vi "Periodic Tasks.vi"(8 "error constant":errorcluster) -> ()   [LabVIEW 2017]
doc: "This VI runs in parallel to other tasks. It can contain as many user-defined periodic loops as you need. These can carry out PID or other sorts of timed response."
uses:
  <vilib>/Rock Robotics/WPI/ThirdParty/Phoenix-LabVIEW/Motor Controller/Controls/CTRE_Phoenix_MotorControl_StatusFrameEnhanced.ctl
  <vilib>/Rock Robotics/WPI/ThirdParty/Phoenix-LabVIEW/Motor Controller/Controls/CTRE_Phoenix_MotorControl_TrajectoryPointTimeDur.ctl
  <vilib>/Rock Robotics/WPI/ThirdParty/Phoenix-LabVIEW/Controls/CTRE_Phoenix_Params.ctl
  <vilib>/Rock Robotics/WPI/ThirdParty/Phoenix-LabVIEW/Motor Controller/Controls/CTRE_Phoenix_MotorControl_ControlMode.ctl
  <vilib>/Rock Robotics/WPI/Utilities/WPI_GetSetVariantRefNum.vi
  Constants.vi
  SelectedMotionProfileMode.vi
  <vilib>/Utility/file.llb/Read Delimited Spreadsheet (DBL).vi
panel:
  out "Mot Prof  Is Under Run":bool
  out "Mot Prof  Has Under Run":bool
  out "Mot Prof Active Is Last":bool
  out "Mot Prof Active Is Valid":bool
  out "Top Mot Prof Count":i32
  out "Mot Prof Active Velocity":dbl
  out "Mot Prof Active Position":dbl
  out "Loop Time":u32
  out "Btm Mot Prof Count":i32
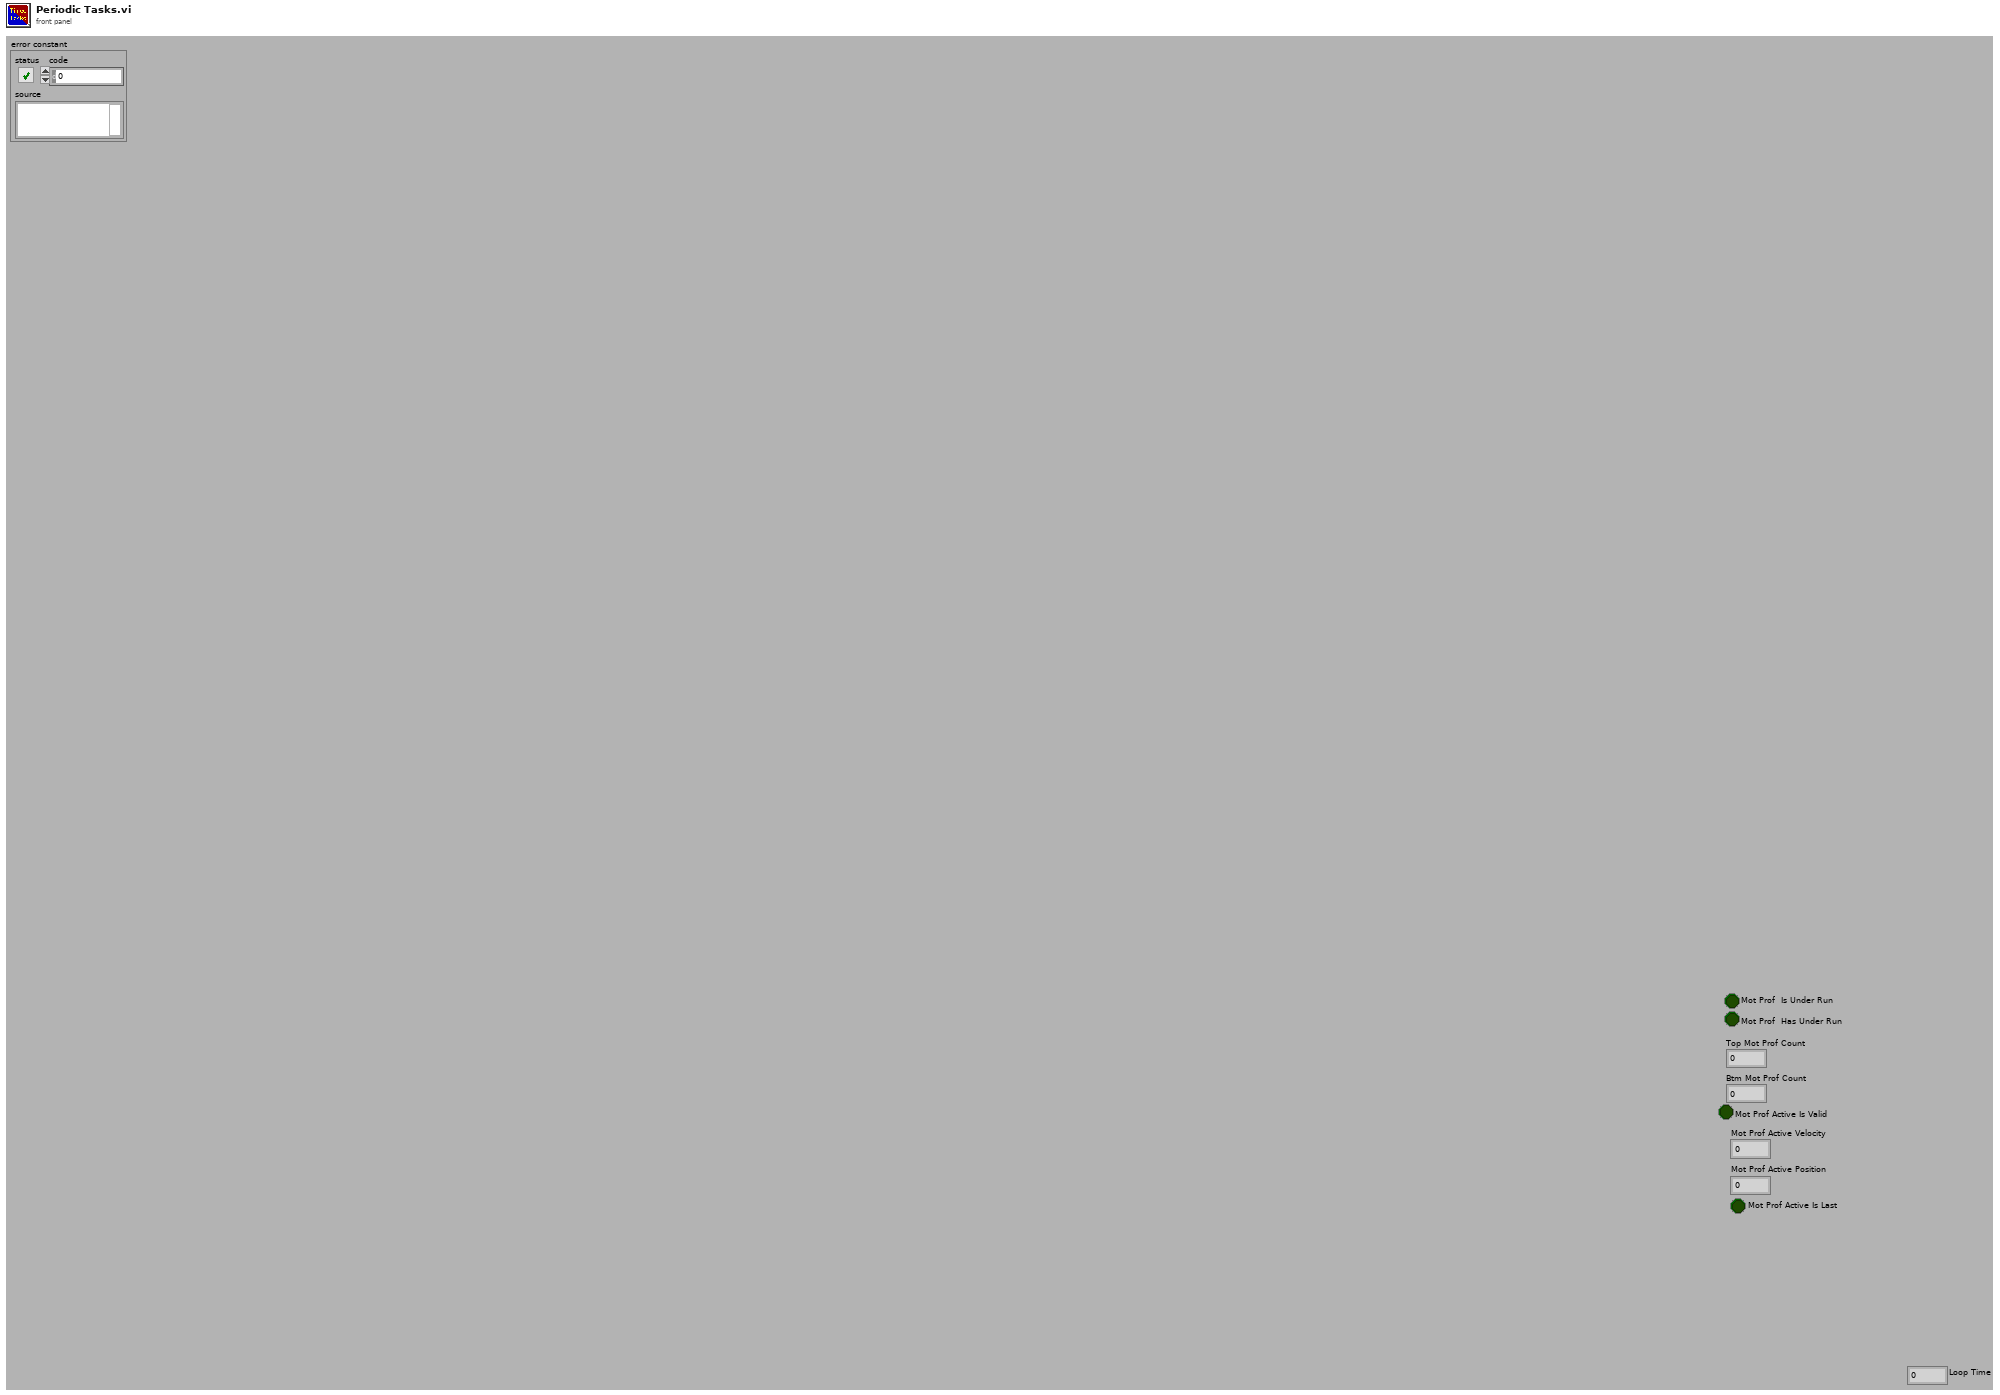
[diagram p1: front panel]
types:
  T1 = typedef "CTRE_Phoenix_MotorControl_StatusFrameEnhanced.ctl" = u16
  T2 = enum16{"One_Axis_PercentOutput", "Two_Axis_PercentOutput", "One_Axix_Position", "One_Axis_Position_CustomFeedFwd", "Two_Axis_Position", "One_Axis_Velocity", "One_Axis_Velocity_CustomFeedFwd", "Two_Axis_Velocity", "One_Axis_MotionMagic", "One_Axis_MotionMagic_CustomFeedFwd", "Two_Axis_MotionMagic", "One_Axis_MotionProfile", "One_Axis_MotionProfile_CustomFeedFwd", "Two_Axis_MotionProfile", "Two_Axis_MotionProfile_CustomFeedFwd"}
  T3 = typedef "WPI_MotorControlDeviceRef.ctl" = cluster{"DeviceStatus":errorcluster, "Type":T4, "PWM":cluster{"PWM Channel":T5, "DeadBand":T6}, "CAN":cluster{"Device Number":u8, "SetOutput VI Ref":variant, "GetOutput VI Ref":variant, "Enable VI Ref":variant, "Disable VI Ref":variant, "Data":variant}, "Invert":bool, "DIO PWM":cluster{"PWM \"Enable\" Channel":T5, "DIOChannel":T7, "PWM Rate":dbl}}
  T4 = typedef "WPI_MotorControlType.ctl" = enum16{"PWM", "CAN", "DIO PWM"}
  T5 = typedef "FPGA_DIOPWMChannel.ctl" = enum8{"PWM 0", "PWM 1", "PWM 2", "PWM 3", "PWM 4", "PWM 5", "PWM 6", "PWM 7", "PWM 8", "PWM 9", "PWM MXP 0", "PWM MXP 1", "PWM MXP 2", "PWM MXP 3", "PWM MXP 4", "PWM MXP 5", "PWM MXP 6", "PWM MXP 7", "PWM MXP 8", "PWM MXP 9", "Invalid"}
  T6 = typedef "WPI_PWMDeadband.ctl" = cluster{"Name":string, "maxPositivePwm":i32, "minPositivePwm":i32, "centerPwm":i32, "maxNegativePwm":i32, "minNegativePwm":i32, "angularRange":u16}
  T7 = typedef "FPGA_DIOChannel.ctl" = enum8{"DIO 0", "DIO 1", "DIO 2", "DIO 3", "DIO 4", "DIO 5", "DIO 6", "DIO 7", "DIO 8", "DIO 9", "DIO MXP 0", "DIO MXP 1", "DIO MXP 2", "DIO MXP 3", "DIO MXP 4", "DIO MXP 5", "DIO MXP 6", "DIO MXP 7", "DIO MXP 8", "DIO MXP 9", "DIO MXP 10", "DIO MXP 11", "DIO MXP 12", "DIO MXP 13", "DIO MXP 14", "DIO MXP 15", "SPI Port CS1", "SPI Port CS2", "SPI Port CS3", "SPI Port MISO", "SPI Port MOSI", "Invalid"}
  T8 = typedef "CTRE_PigeonIMU_DeviceRef.ctl" = cluster{"DeviceStatus":errorcluster, "Device Number":u8, "Type":T9, "Device ID":u32, "Handle":u64, "UsageFrame":u32, "Library Path":path}
  T9 = typedef "CTRE_PigeonIMU_ConnectionType.ctl" = u32
  T10 = typedef "WPI_JoystickDevRef.ctl" = cluster{"Device":T11}
  T11 = typedef "WPI_JoystickDeviceEnum.ctl" = enum16{"USB 0", "USB 1", "USB 2", "USB 3", "USB 4", "USB 5"}
  T12 = enum16{"DemandType_Neutral", "DemandType_AuxPID", "DemandType_ArbitraryFeedForward"}
  T13 = enum16{"FollowerType_PercentOutput", "FollowerType_AuxOutput1"}
  T14 = typedef "CTRE_Phoenix_Params.ctl" = u16
  T15 = typedef "CTRE_Phoenix_MotorControl_ControlMode.ctl" = u16
  T16 = cluster{"Top Buffer Remaining":i32, "Top Buffer Count":i32, "Bottom Buffer Count":i32, "Has Underrun?":bool, "Is Underrun?":bool, "Active Point Valid?":bool, "Is Last?":bool, "Profile Slot Select 0":i32, "Output Enable":i32, "Time Duration (ms)":i32, "Profile Slot Select 1":i32}
  T17 = typedef "CTRE_Phoenix_MotorControl_TrajectoryPointTimeDur.ctl" = i32
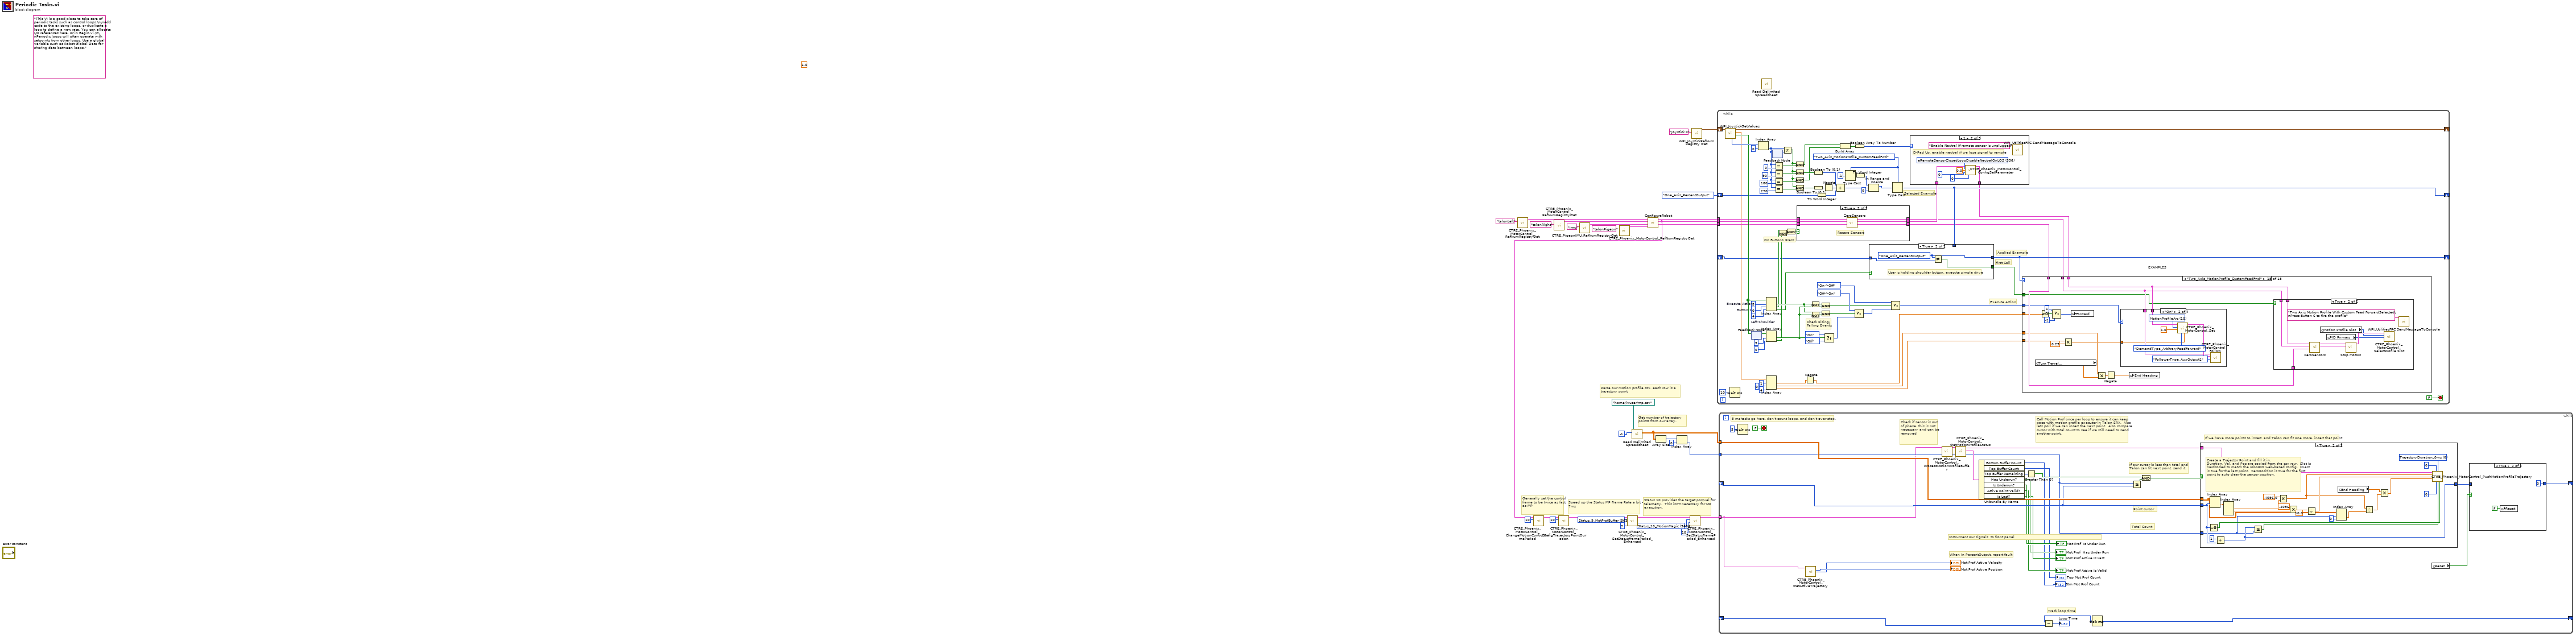
[diagram p0: block diagram]
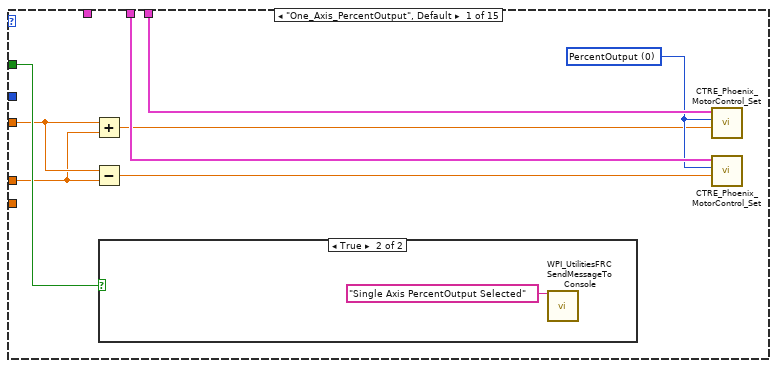
[diagram p4: hidden frame]
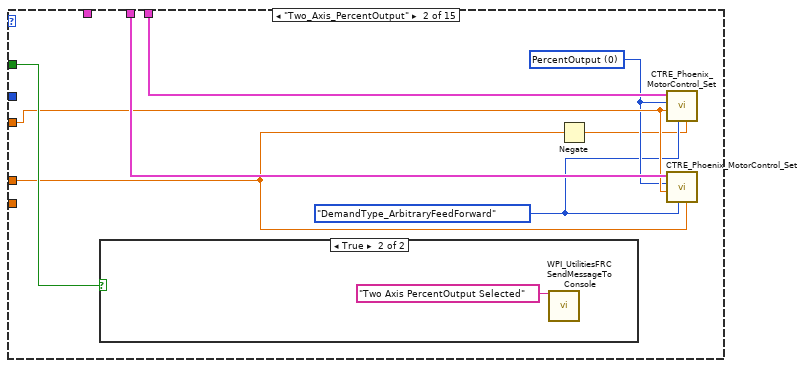
[diagram p6: hidden frame]
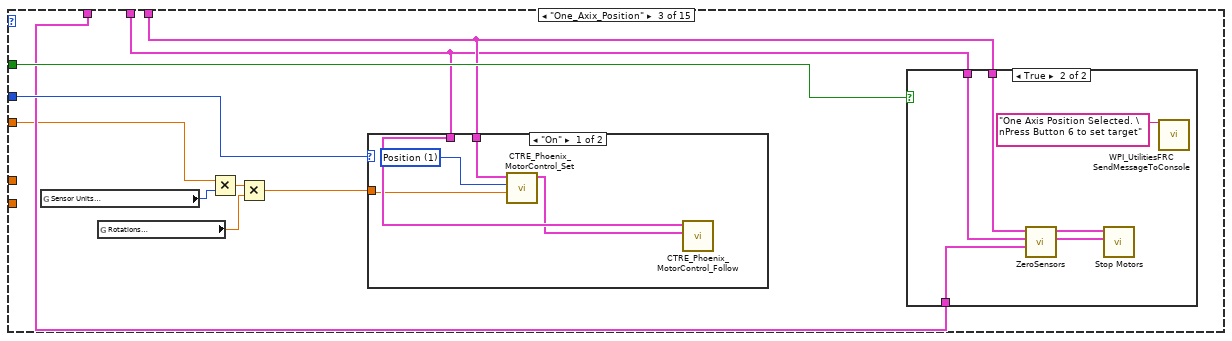
[diagram p8: hidden frame]
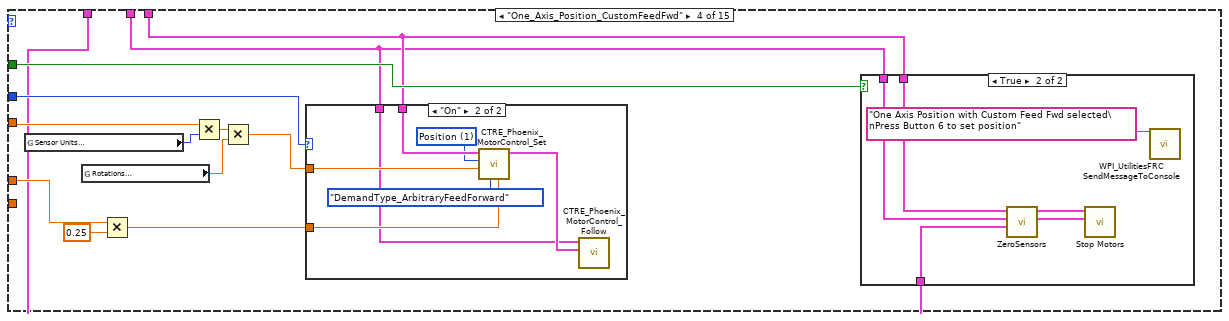
[diagram p11: hidden frame]
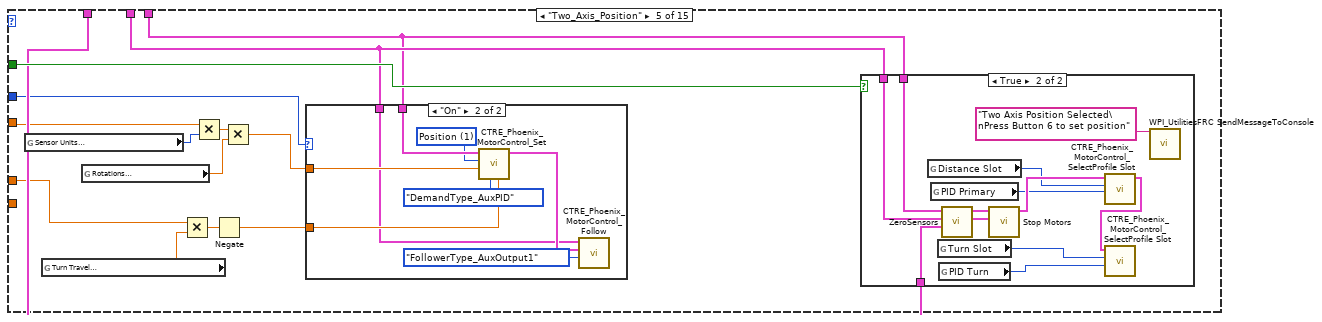
[diagram p14: hidden frame]
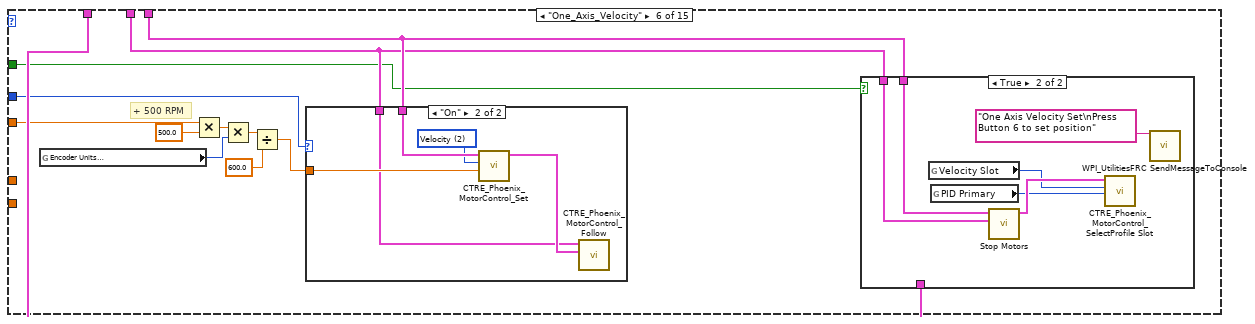
[diagram p17: hidden frame]
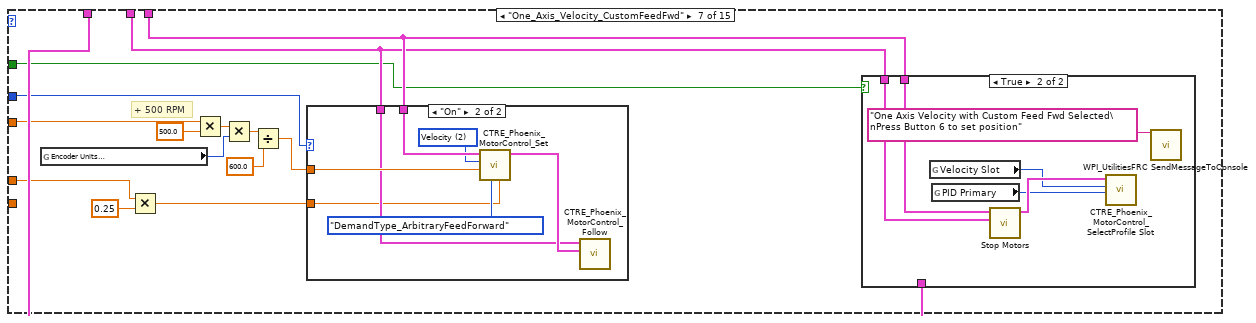
[diagram p20: hidden frame]
diagram:
  w9 = T1 5696 items=["Status_1_General"=5120, "Status_2_Feedback0"=5184, "Status_3_Quadrature"=5248, "Status_4_AinTempVbat"=5312, "Status_6_Misc"=5440, "Status_7_CommStatus"=5504, "Status_8_PulseWidth"=5568, "Status_9_MotProfBuffer"=5632, "Status_10_MotionMagic"=5696, "Status_11_UartGadgeteer"=5760, "Status_12_Feedback1"=5824, "Status_13_Base_PIDF0"=5888, "Status_14_Turn_PIDF1"=5952, "Status_15_FirmwareApiStatus"=6016] ("Status Frame")
  w11 = T1 5632 items=["Status_1_General"=5120, "Status_2_Feedback0"=5184, "Status_3_Quadrature"=5248, "Status_4_AinTempVbat"=5312, "Status_6_Misc"=5440, "Status_7_CommStatus"=5504, "Status_8_PulseWidth"=5568, "Status_9_MotProfBuffer"=5632, "Status_10_MotionMagic"=5696, "Status_11_UartGadgeteer"=5760, "Status_12_Feedback1"=5824, "Status_13_Base_PIDF0"=5888, "Status_14_Turn_PIDF1"=5952, "Status_15_FirmwareApiStatus"=6016] ("Status Frame")
  (unwired) 1.0 ("Forward Peak Percent Output")
  (unwired) "This VI is a good place to take care of periodic tasks such as control loops.\n\nAdd code to the existing loops, or duplicate a loop to define a new rate. You can allocate I/O references here, or in Begin.vi.\n\nPeriodic loops will often operate with setpoints from other loops. Use a global variable such as Robot Global Data for sharing data between loops."
  # "Generally set the control frame to be twice as fast as MP"
  # "Status 10 provides the target pos/vel for telemetry.  This isn't necessary for MP execution."
  # "Speed up the Status MP Frame Rate a bit - 7ms"
  # "Get number of trajectory points from our array."
  # "Parse our motion profile csv, each row is a trajectory point"
  n1 = call <vilib>:"CTRE_Phoenix_MotorControl_RefNumRegistryGet.vi"("refnum name"="talonLeft") -> ("PhoenixMotorControlDevRef"=w23:T3)  [unwired: 9 in, 1 out]
  n2 = call <vilib>:"CTRE_Phoenix_MotorControl_RefNumRegistryGet.vi"("refnum name"="talonRight") -> ("PhoenixMotorControlDevRef"=w24:T3)  [unwired: 9 in, 1 out]
  n3 = call <vilib>:"CTRE_PigeonIMU_RefNumRegistryGet.vi"("refnum name"="imu") -> ("PigeonIMUDevRef"=w19:T8)  [unwired: 9 in, 1 out]
  n4 = call <vilib>:"CTRE_Phoenix_MotorControl_RefNumRegistryGet.vi"("refnum name"="talonPigeon") -> ("PhoenixMotorControlDevRef"=w18:T3)  [unwired: 9 in, 1 out]
  n5 = call-poly <vilib>:"Read Delimited Spreadsheet.vi"("file path (dialog if empty)"=path "/home/lvuser/mp.csv" ("file path (use dialog)"), "number of rows (all:-1)"=-1) -> ("all rows"=w13:dbl[][])  [unwired: 8 in, 5 out]
  n6 = call "ConfigureRobot.vi"("Pigeon Talon"=w18, "Pigeon"=w19, "Right Side"=w24, "Left Side"=w23) -> ("Pigeon"=w20:T8, "Right Side"=w4:T3, "Left Side"=w21:T3)  [unwired: 5 in]
  n7 = call <vilib>:"CTRE_Phoenix_MotorControl_ChangeMotionControlFramePeriod.vi"("periodMs"=10, "PhoenixMotorControlDevRef"=w4) -> ("PhoenixMotorControlDevRef"=w3:T3)  [unwired: 8 in, 1 out]
  n8 = call <vilib>:"CTRE_Phoenix_MotorControl_ConfigTrajectoryPointDuration.vi"("durationMs"=10, "PhoenixMotorControlDevRef"=w3) -> ("PhoenixMotorControlDevRef"=w2:T3)  [unwired: 8 in, 1 out]
  n9 = call <vilib>:"CTRE_Phoenix_MotorControl_SetStatusFramePeriod_Enhanced.vi"("periodMs"=7, "Status Frame"=w11, "PhoenixMotorControlDevRef"=w2) -> ("PhoenixMotorControlDevRef"=w7:T3)  [unwired: 7 in, 1 out]
  n10 = Array Size(array=w13) -> (size(s)=w14:i32[])
  n11 = Index Array(array=w14, index=0) -> (element=w12:i32)
  n12 = call <vilib>:"CTRE_Phoenix_MotorControl_SetStatusFramePeriod_Enhanced.vi"("periodMs"=10, "Status Frame"=w9, "PhoenixMotorControlDevRef"=w7) -> ("PhoenixMotorControlDevRef"=w5:T3)  [unwired: 7 in, 1 out]
  n13 = call <vilib>:"WPI_JoystickRefNum Registry Get.vi"("refnum name"="Joystick 0") -> ("JoystickDevRef"=w29:T10)  [unwired: 1 in, 9 out]
  n14 = while {
    shift-right: [w106] -> _
    shift-left: w29 -> [w107]
    shift-right: [w56] -> _
    shift-left: T2."One_Axis_PercentOutput" -> [w55]
    tunnel: w21 -> [w70]
    tunnel: w4 -> [w69]
    tunnel: w20 -> [w68]
    shift-right: [w57] -> _
    shift-left: _ -> [w58]
    stop <- FALSE stop-if-true
    w49 = T2."Two_Axis_MotionProfile_CustomFeedFwd"
    w60 = 4  # Left Shoulder
    w66 = 0  # Button 1
    w84 = 5  # Execute Action
    # "Execute Action"
    # "Check Rising/\nFalling Events"
    # "First Call"
    # "Applied Example"
    # "On Button1 Press"
    # "Selected Example"
    n15 = call <vilib>:"WPI_JoystickGetValues.vi"("JoystickDevRef"=w107) -> ("Buttons"=w86:bool[], "Axes"=w44:dbl[], "JoystickDevRef"=w106:T10, "POVs"=w105:i16[])  [unwired: 6 in, 1 out]
    n16 = Wait (ms)(milliseconds to wait=u32 10) -> ()  [unwired: 1 out]
    n17 = feedback #1() -> (w85:bool[])  [unwired: 1 in]
    n18 = feedback-in #1(w86) -> ()
    n19 = Index Array(array=w105, index=0) -> (element=w98:i16)
    n20 = Index Array(array=w86, index #1=w84, index #2=w66, index #3=w60) -> (element #1=w77:bool, element #2=w63:bool, element #3=w59:bool)
    n21 = Index Array(array=w85, index #1=5 ("index"), index #2=0 ("index")) -> (element #1=w78:bool, element #2=w61:bool)
    n22 = Index Array(array=w44, index #1=1 ("index"), index #2=0 ("index"), index #3=4 ("index")) -> (element #1=w32:dbl, element #2=w41:dbl, element #3=w33:dbl)
    n23 = feedback #2() -> (w99:i16)  [unwired: 1 in]
    n24 = feedback-in #2(w98) -> ()
    n25 = Equal?(x=w98, y=i16 0) -> (x = y?=w97:bool)
    n26 = Equal?(x=w98, y=i16 90) -> (x = y?=w96:bool)
    n27 = Equal?(x=w98, y=i16 180) -> (x = y?=w95:bool)
    n28 = Equal?(x=w98, y=i16 270) -> (x = y?=w94:bool)
    n29 = Not(x=w61) -> (.not. x?=w62:bool)
    n30 = Not Equal?(x=w98, y=w99) -> (x != y?=w93:bool)
    n31 = And(x=w63, y=w62) -> (x .and. y?=w64:bool)
    n32 = And(x=w93, y=w97) -> (x .and. y?=w88:bool)
    n33 = And(x=w93, y=w96) -> (x .and. y?=w91:bool)
    n34 = And(x=w93, y=w95) -> (x .and. y?=w87:bool)
    n35 = And(x=w93, y=w94) -> (x .and. y?=w92:bool)
    n36 = case shown="True" w64 {
      tunnel: w70 -> [w542 w544]
      tunnel: w69 -> [w543 w545]
      tunnel: w68 -> [w541 w546]
      tunnel: [w543 w548] -> w67
      tunnel: [w542 w549] -> w40
      tunnel: [w541 w547] -> w35
      frame False {
        # "Do Nothing"
      }
      frame True {
        # "Rezero Sensors"
        n37 = call "ZeroSensors.vi"("Pigeon"=w546, "Talon 2"=w545, "Talon 1"=w544) -> ("Pigeon"=w547:T8, "Talon 2"=w548:T3, "Talon 1"=w549:T3)  [unwired: 6 in]
      }
    }
    n38 = Negate(x=w32) -> (-x=w31:dbl)
    n39 = Not(x=w77) -> (.not. x?=w79:bool)
    n40 = Not(x=w78) -> (.not. x?=w80:bool)
    n41 = Boolean To (0,1)(Boolean=w91) -> (0, 1=w38:i16)
    n42 = Boolean To (0,1)(Boolean=w92) -> (0, 1=w36:i16)
    n43 = To Word Integer(number=w55) -> (16bit integer=w54:i16)
    n44 = And(x=w79, y=w78) -> (x .and. y?=w71:bool)
    n45 = And(x=w77, y=w80) -> (x .and. y?=w72:bool)
    n46 = Negate(x=w36) -> (-x=w37:i16)
    n47 = Select(t=enum16{"Off->On", "On->Off", "On", "Off"}."On", s=w78, f=enum16{"Off->On", "On->Off", "On", "Off"}."Off") -> (s? t:f=w76:enum16{"Off->On", "On->Off", "On", "Off"})
    n48 = Compound Arithmetic op=ADD(w38, w37, w54) -> (w53:i16)
    n49 = Build Array(w88, w87) -> (w89:bool[])
    n50 = Type Cast(type=w49, x=i16 -1 ("lower limit")) -> (*(type *) &x=w47:T2)
    n51 = Select(t=enum16{"Off->On", "On->Off", "On", "Off"}."Off->On", s=w72, f=w76) -> (s? t:f=w75:enum16{"Off->On", "On->Off", "On", "Off"})
    n52 = Boolean Array To Number(Boolean array=w89) -> (number=w90:u32)
    n53 = To Word Integer(number=w47) -> (16bit integer=w48:i16)
    n54 = In Range and Coerce(upper limit=w48, x=w53, lower limit=i16 0) -> (coerced(x)=w51:i16)  [unwired: 1 out]
    n55 = Select(t=enum16{"Off->On", "On->Off", "On", "Off"}."On->Off", s=w71, f=w75) -> (s? t:f=w45:enum16{"Off->On", "On->Off", "On", "Off"})
    n56 = Type Cast(type=w49, x=w51) -> (*(type *) &x=w56:T2)
    n57 = case shown="True" w59 {
      tunnel: w58 -> [w535 w540]
      tunnel: [w537 w539] -> w46
      tunnel: [w536 w538] -> w57
      tunnel: w56 -> [w536 _]
      frame False {
        # "User is not holding shoulder button, use applied example"
        n58 = Not Equal?(x=w536, y=w535) -> (x != y?=w537:bool)
      }
      frame True {
        w538 = T2."One_Axis_PercentOutput"
        # "User is holding shoulder button, execute simple drive"
        n59 = Not Equal?(x=w538, y=w540) -> (x != y?=w539:bool)
      }
    }
    n60 = case shown="1" w90 {
      tunnel: w67 -> [w550 w552 w564]
      tunnel: [w550 w553 w563] -> w39
      frame 0, Default {
        # "Nothing Pressed"
      }
      frame 1 {
        w557 = T14 336 items=["eOnBoot_BrakeMode"=31, "eQuadFilterEn"=91, "eQuadIdxPolarity"=108, "eClearPositionOnIdx"=100, "eMotionProfileHasUnderrunErr"=119, "eMotionProfileTrajectoryPointDurationMs"=120, "eClearPosOnLimitF"=144, "eClearPosOnLimitR"=145, "eStatusFramePeriod"=300, "eOpenLoopRamp"=301, "eClosedLoopRamp"=302, "eNeutralDeadband"=303, "ePeakPosOutput"=305, "eNominalPosOutput"=306, "ePeakNegOutput"=307, "eNominalNegOutput"=308, "eProfileParamSlot_P"=310, "eProfileParamSlot_I"=311, "eProfileParamSlot_D"=312, "eProfileParamSlot_F"=313, "eProfileParamSlot_IZone"=314, "eProfileParamSlot_AllowableErr"=315, "eProfileParamSlot_MaxIAccum"=316, "eClearPositionOnLimitF"=320, "eClearPositionOnLimitR"=321, "eClearPositionOnQuadIdx"=322, "eSampleVelocityPeriod"=325, "eSampleVelocityWindow"=326, "eFeedbackSensorType"=330, "eSelectedSensorPosition"=331, "eFeedbackNotContinuous"=332, "eRemoteSensorSource"=333, "eRemoteSensorDeviceID"=334, "eSensorTerm"=335, "eRemoteSensorClosedLoopDisableNeutralOnLOS"=336, "eForwardSoftLimitThreshold"=340, "eReverseSoftLimitThreshold"=341, "eForwardSoftLimitEnable"=342, "eReverseSoftLimitEnable"=343, "eNominalBatteryVoltage"=350, "eBatterVoltageFilterSize"=351, "eContinuousCurrentLimitAmps"=360, "eContinuousCurrentLimitMs"=361, "ePeakCurrentLimitAmps"=362, "eClosedLoopIAccum"=370, "eCustomParam"=380, "eStickyFaults"=390, "eAnalogPosition"=400, "eQuadraturePosition"=401, "ePulseWidthPosition"=402, "eMotMag_Accel"=410, "eMotMag_VelCruise"=411, "eLimitSwitchSource"=421, "eLimitSwitchNormClosedAndDis"=422, "eLimitSwitchDisabledNeutralOnLOS"=423, "eLimitSwitchRemoteDevID"=424] ("Parameter")
        # "D-Pad Up, enable neutral if we lose signal to remote"
        n61 = call <vilib>:"CTRE_Phoenix_MotorControl_ConfigSetParameter.vi"("PhoenixMotorControlDevRef"=w552, "Parameter"=w557, "value"=0.0, "subValue"=u8 0, "ordinal"=0) -> ("PhoenixMotorControlDevRef"=w553:T3)  [unwired: 9 in, 1 out]
        n62 = call <vilib>:"WPI_UtilitiesFRC SendMessageToConsole.vi"("Message"="Enable Neutral if remote sensor is unplugged") -> ()  [unwired: 14 in, 1 out]
      }
      frame 2 {
        w562 = T14 336 items=["eOnBoot_BrakeMode"=31, "eQuadFilterEn"=91, "eQuadIdxPolarity"=108, "eClearPositionOnIdx"=100, "eMotionProfileHasUnderrunErr"=119, "eMotionProfileTrajectoryPointDurationMs"=120, "eClearPosOnLimitF"=144, "eClearPosOnLimitR"=145, "eStatusFramePeriod"=300, "eOpenLoopRamp"=301, "eClosedLoopRamp"=302, "eNeutralDeadband"=303, "ePeakPosOutput"=305, "eNominalPosOutput"=306, "ePeakNegOutput"=307, "eNominalNegOutput"=308, "eProfileParamSlot_P"=310, "eProfileParamSlot_I"=311, "eProfileParamSlot_D"=312, "eProfileParamSlot_F"=313, "eProfileParamSlot_IZone"=314, "eProfileParamSlot_AllowableErr"=315, "eProfileParamSlot_MaxIAccum"=316, "eClearPositionOnLimitF"=320, "eClearPositionOnLimitR"=321, "eClearPositionOnQuadIdx"=322, "eSampleVelocityPeriod"=325, "eSampleVelocityWindow"=326, "eFeedbackSensorType"=330, "eSelectedSensorPosition"=331, "eFeedbackNotContinuous"=332, "eRemoteSensorSource"=333, "eRemoteSensorDeviceID"=334, "eSensorTerm"=335, "eRemoteSensorClosedLoopDisableNeutralOnLOS"=336, "eForwardSoftLimitThreshold"=340, "eReverseSoftLimitThreshold"=341, "eForwardSoftLimitEnable"=342, "eReverseSoftLimitEnable"=343, "eNominalBatteryVoltage"=350, "eBatterVoltageFilterSize"=351, "eContinuousCurrentLimitAmps"=360, "eContinuousCurrentLimitMs"=361, "ePeakCurrentLimitAmps"=362, "eClosedLoopIAccum"=370, "eCustomParam"=380, "eStickyFaults"=390, "eAnalogPosition"=400, "eQuadraturePosition"=401, "ePulseWidthPosition"=402, "eMotMag_Accel"=410, "eMotMag_VelCruise"=411, "eLimitSwitchSource"=421, "eLimitSwitchNormClosedAndDis"=422, "eLimitSwitchDisabledNeutralOnLOS"=423, "eLimitSwitchRemoteDevID"=424] ("Parameter")
        # "D-Pad Up, disable neutral if we lose signal to remote"
        n63 = call <vilib>:"CTRE_Phoenix_MotorControl_ConfigSetParameter.vi"("PhoenixMotorControlDevRef"=w564, "Parameter"=w562, "value"=1.0, "subValue"=u8 0, "ordinal"=0) -> ("PhoenixMotorControlDevRef"=w563:T3)  [unwired: 9 in, 1 out]
        n64 = call <vilib>:"WPI_UtilitiesFRC SendMessageToConsole.vi"("Message"="Disable Neutral if remote sensor is unplugged") -> ()  [unwired: 14 in, 1 out]
      }
    }
    n65 = case "EXAMPLES" shown="\"Two_Axis_MotionProfile_CustomFeedFwd\"" w57 {
      tunnel: w46 -> [w115 w126 w137 w161 w184 w216 w237 w269 w297 w323 w343 w384 w416 w460 w497]
      tunnel: w45 -> [_ _ w136 w160 w180 w215 w236 w268 w296 w324 w349 w383 w415 w456 w496]
      tunnel: w31 -> [w113 w123 w128 w156 w179 w214 w235 w267 w295 w325 w348 w382 w414 w455 w495]
      tunnel: w41 -> [w112 w120 _ w155 w178 _ w234 w266 _ w319 w347 _ _ w454 w494]
      tunnel: w40 -> [w116 w124 w130 w150 w182 w218 w239 w264 w298 w321 w345 w386 w418 w458 w499]
      tunnel: w39 -> [w117 w125 w131 w151 w181 w219 w240 w263 w300 w320 w344 w387 w419 w457 w500]
      tunnel: w35 -> [_ _ w129 w149 w183 w217 w238 w265 w299 w322 w346 w385 w417 w459 w498]
      tunnel: w33 -> [_ _ _ _ _ _ _ _ _ _ _ _ w411 _ w493]
      frame "One_Axis_PercentOutput", Default {
        w114 = T15 0 items=["PercentOutput"=0, "Position"=1, "Velocity"=2, "Current"=3, "Follower"=5, "MotionProfile"=6, "MotionMagic"=7, "MotionMagicArc"=8, "MotionProfileArc"=10, "Disabled"=15] ("Control Mode")
        n66 = Add(x=w113, y=w112) -> (x+y=w110:dbl)
        n67 = Subtract(x=w113, y=w112) -> (x-y=w111:dbl)
        n68 = case shown="True" w115 {
          frame False {
          }
          frame True {
            n69 = call <vilib>:"WPI_UtilitiesFRC SendMessageToConsole.vi"("Message"="Single Axis PercentOutput Selected") -> ()  [unwired: 14 in, 1 out]
          }
        }
        n70 = call <vilib>:"CTRE_Phoenix_MotorControl_Set.vi"("Output"=w110, "Control Mode"=w114, "PhoenixMotorControlDevRef"=w117) -> ()  [unwired: 7 in, 2 out]
        n71 = call <vilib>:"CTRE_Phoenix_MotorControl_Set.vi"("Output"=w111, "Control Mode"=w114, "PhoenixMotorControlDevRef"=w116) -> ()  [unwired: 7 in, 2 out]
      }
      frame "Two_Axis_PercentOutput" {
        w121 = T12."DemandType_ArbitraryFeedForward" ("DemandType")
        w122 = T15 0 items=["PercentOutput"=0, "Position"=1, "Velocity"=2, "Current"=3, "Follower"=5, "MotionProfile"=6, "MotionMagic"=7, "MotionMagicArc"=8, "MotionProfileArc"=10, "Disabled"=15] ("Control Mode")
        n72 = case shown="True" w126 {
          frame False {
          }
          frame True {
            n73 = call <vilib>:"WPI_UtilitiesFRC SendMessageToConsole.vi"("Message"="Two Axis PercentOutput Selected") -> ()  [unwired: 14 in, 1 out]
          }
        }
        n74 = Negate(x=w120) -> (-x=w119:dbl)
        n75 = call <vilib>:"CTRE_Phoenix_MotorControl_Set.vi"("Demand1"=w119, "DemandType"=w121, "Output"=w123, "Control Mode"=w122, "PhoenixMotorControlDevRef"=w125) -> ()  [unwired: 5 in, 2 out]
        n76 = call <vilib>:"CTRE_Phoenix_MotorControl_Set.vi"("Demand1"=w120, "DemandType"=w121, "Output"=w123, "Control Mode"=w122, "PhoenixMotorControlDevRef"=w124) -> ()  [unwired: 5 in, 2 out]
      }
      frame "One_Axix_Position" {
        n77 = global read "Constants.vi" "Sensor Units\nPer Rotation"() -> (w134:i32)
        n78 = global read "Constants.vi" "Rotations\nTo Travel"() -> (w133:dbl)
        n79 = Multiply(x=w128, y=w134) -> (x*y=w135:dbl)
        n80 = Multiply(x=w135, y=w133) -> (x*y=w132:dbl)
        n81 = case shown="\"On\"" w136 {
          tunnel: w132 -> [w138 _]
          tunnel: w131 -> [w142 _]
          tunnel: w130 -> [w140 _]
          frame "On" {
            w141 = T15 1 items=["PercentOutput"=0, "Position"=1, "Velocity"=2, "Current"=3, "Follower"=5, "MotionProfile"=6, "MotionMagic"=7, "MotionProfileArc"=10, "Disabled"=15] ("Control Mode")
            n82 = call <vilib>:"CTRE_Phoenix_MotorControl_Set.vi"("Output"=w138, "Control Mode"=w141, "PhoenixMotorControlDevRef"=w142) -> ("PhoenixMotorControlDevRef"=w139:T3)  [unwired: 7 in, 1 out]
            n83 = call <vilib>:"CTRE_Phoenix_MotorControl_Follow.vi"("Master Controller to Follow"=w139, "PhoenixMotorControlDevRef"=w140) -> ()  [unwired: 8 in, 2 out]
          }
          frame Default {
          }
        }
        n84 = case shown="True" w137 {
          tunnel: w131 -> [_ w147]
          tunnel: w130 -> [_ w146]
          tunnel: w129 -> [_ w145]
          frame False {
          }
          frame True {
            n85 = call "ZeroSensors.vi"("Pigeon"=w145, "Talon 2"=w146, "Talon 1"=w147) -> ("Talon 2"=w143:T3, "Talon 1"=w144:T3)  [unwired: 6 in, 1 out]
            n86 = call "Stop Motors.vi"("Talon SRX 2"=w143, "Talon SRX 1"=w144) -> ()  [unwired: 8 in, 2 out]
            n87 = call <vilib>:"WPI_UtilitiesFRC SendMessageToConsole.vi"("Message"="One Axis Position Selected. \nPress Button 6 to set target") -> ()  [unwired: 14 in, 1 out]
          }
        }
      }
      frame "One_Axis_Position_CustomFeedFwd" {
        n88 = global read "Constants.vi" "Sensor Units\nPer Rotation"() -> (w158:i32)
        n89 = global read "Constants.vi" "Rotations\nTo Travel"() -> (w157:dbl)
        n90 = Multiply(x=w155, y=0.25) -> (x*y=w152:dbl)
        n91 = Multiply(x=w156, y=w158) -> (x*y=w159:dbl)
        n92 = Multiply(x=w159, y=w157) -> (x*y=w153:dbl)
        n93 = case shown="\"On\"" w160 {
          tunnel: w151 -> [_ w168]
          tunnel: w150 -> [_ w162]
          tunnel: w152 -> [_ w164]
          tunnel: w153 -> [_ w166]
          frame Default {
          }
          frame "On" {
            w167 = T15 1 items=["PercentOutput"=0, "Position"=1, "Velocity"=2, "Current"=3, "Follower"=5, "MotionProfile"=6, "MotionMagic"=7, "MotionProfileArc"=10, "Disabled"=15] ("Control Mode")
            n94 = call <vilib>:"CTRE_Phoenix_MotorControl_Set.vi"("Demand1"=w164, "DemandType"=T12."DemandType_ArbitraryFeedForward", "Output"=w166, "Control Mode"=w167, "PhoenixMotorControlDevRef"=w168) -> ("PhoenixMotorControlDevRef"=w163:T3)  [unwired: 5 in, 1 out]
            n95 = call <vilib>:"CTRE_Phoenix_MotorControl_Follow.vi"("Master Controller to Follow"=w163, "PhoenixMotorControlDevRef"=w162) -> ()  [unwired: 8 in, 2 out]
          }
        }
        n96 = case shown="True" w161 {
          tunnel: w151 -> [_ w171]
          tunnel: w150 -> [_ w170]
          tunnel: w149 -> [_ w169]
          frame False {
          }
          frame True {
            n97 = call "ZeroSensors.vi"("Pigeon"=w169, "Talon 2"=w170, "Talon 1"=w171) -> ("Talon 2"=w172:T3, "Talon 1"=w173:T3)  [unwired: 6 in, 1 out]
            n98 = call "Stop Motors.vi"("Talon SRX 2"=w172, "Talon SRX 1"=w173) -> ()  [unwired: 8 in, 2 out]
            n99 = call <vilib>:"WPI_UtilitiesFRC SendMessageToConsole.vi"("Message"="One Axis Position with Custom Feed Fwd selected\nPress Button 6 to set position") -> ()  [unwired: 14 in, 1 out]
          }
        }
      }
      frame "Two_Axis_Position" {
        n100 = global read "Constants.vi" "Sensor Units\nPer Rotation"() -> (w187:i32)
        n101 = global read "Constants.vi" "Turn Travel\nUnits Per Rotation"() -> (w177:dbl)
        n102 = global read "Constants.vi" "Rotations\nTo Travel"() -> (w186:dbl)
        n103 = Multiply(x=w178, y=w177) -> (x*y=w176:dbl)
        n104 = Multiply(x=w179, y=w187) -> (x*y=w188:dbl)
        n105 = Negate(x=w176) -> (-x=w175:dbl)
        n106 = Multiply(x=w188, y=w186) -> (x*y=w185:dbl)
        n107 = case shown="\"On\"" w180 {
          tunnel: w181 -> [_ w196]
          tunnel: w182 -> [_ w190]
          tunnel: w175 -> [_ w192]
          tunnel: w185 -> [_ w194]
          frame Default {
          }
          frame "On" {
            w195 = T15 1 items=["PercentOutput"=0, "Position"=1, "Velocity"=2, "Current"=3, "Follower"=5, "MotionProfile"=6, "MotionMagic"=7, "MotionProfileArc"=10, "Disabled"=15] ("Control Mode")
            n108 = call <vilib>:"CTRE_Phoenix_MotorControl_Set.vi"("Demand1"=w192, "DemandType"=T12."DemandType_AuxPID", "Output"=w194, "Control Mode"=w195, "PhoenixMotorControlDevRef"=w196) -> ("PhoenixMotorControlDevRef"=w191:T3)  [unwired: 5 in, 1 out]
            n109 = call <vilib>:"CTRE_Phoenix_MotorControl_Follow.vi"("FollowerType"=T13."FollowerType_AuxOutput1", "Master Controller to Follow"=w191, "PhoenixMotorControlDevRef"=w190) -> ()  [unwired: 7 in, 2 out]
          }
        }
        n110 = case shown="True" w184 {
          tunnel: w181 -> [_ w205]
          tunnel: w182 -> [_ w204]
          tunnel: w183 -> [_ w203]
          frame False {
          }
          frame True {
            n111 = global read "Constants.vi" "Distance Slot"() -> (w200:i32)
            n112 = global read "Constants.vi" "PID Primary"() -> (w201:i32)
            n113 = global read "Constants.vi" "Turn Slot"() -> (w199:i32)
            n114 = global read "Constants.vi" "PID Turn"() -> (w198:i32)
            n115 = call "ZeroSensors.vi"("Pigeon"=w203, "Talon 2"=w204, "Talon 1"=w205) -> ("Talon 2"=w206:T3, "Talon 1"=w207:T3)  [unwired: 6 in, 1 out]
            n116 = call "Stop Motors.vi"("Talon SRX 2"=w206, "Talon SRX 1"=w207) -> ("Talon SRX 1"=w202:T3)  [unwired: 8 in, 1 out]
            n117 = call <vilib>:"CTRE_Phoenix_MotorControl_SelectProfile Slot.vi"("pidLoopIdx"=w201, "slotIdx"=w200, "PhoenixMotorControlDevRef"=w202) -> ("PhoenixMotorControlDevRef"=w197:T3)  [unwired: 7 in, 1 out]
            n118 = call <vilib>:"CTRE_Phoenix_MotorControl_SelectProfile Slot.vi"("pidLoopIdx"=w198, "slotIdx"=w199, "PhoenixMotorControlDevRef"=w197) -> ()  [unwired: 7 in, 2 out]
            n119 = call <vilib>:"WPI_UtilitiesFRC SendMessageToConsole.vi"("Message"="Two Axis Position Selected\nPress Button 6 to set position") -> ()  [unwired: 14 in, 1 out]
          }
        }
      }
      frame "One_Axis_Velocity" {
        # "+ 500 RPM"
        n120 = global read "Constants.vi" "Encoder Units\nPer Rotation"() -> (w212:i32)
        n121 = Multiply(x=w214, y=500.0) -> (x*y=w220:dbl)
        n122 = Multiply(x=w220, y=w212) -> (x*y=w211:dbl)
        n123 = Divide(x=w211, y=600.0) -> (x/y=w210:dbl)
        n124 = case shown="\"On\"" w215 {
          tunnel: w219 -> [_ w225]
          tunnel: w218 -> [_ w221]
          tunnel: w210 -> [_ w223]
          frame Default {
          }
          frame "On" {
            w224 = T15 2 items=["PercentOutput"=0, "Position"=1, "Velocity"=2, "Current"=3, "Follower"=5, "MotionProfile"=6, "MotionMagic"=7, "MotionProfileArc"=10, "Disabled"=15] ("Control Mode")
            n125 = call <vilib>:"CTRE_Phoenix_MotorControl_Set.vi"("Output"=w223, "Control Mode"=w224, "PhoenixMotorControlDevRef"=w225) -> ("PhoenixMotorControlDevRef"=w222:T3)  [unwired: 7 in, 1 out]
            n126 = call <vilib>:"CTRE_Phoenix_MotorControl_Follow.vi"("Master Controller to Follow"=w222, "PhoenixMotorControlDevRef"=w221) -> ()  [unwired: 8 in, 2 out]
          }
        }
        n127 = case shown="True" w216 {
          tunnel: w219 -> [_ w227]
          tunnel: w218 -> [_ w226]
          tunnel: w217 -> [_ _]
          frame False {
          }
          frame True {
            n128 = global read "Constants.vi" "Velocity Slot"() -> (w228:i32)
            n129 = global read "Constants.vi" "PID Primary"() -> (w229:i32)
            n130 = call "Stop Motors.vi"("Talon SRX 2"=w226, "Talon SRX 1"=w227) -> ("Talon SRX 1"=w230:T3)  [unwired: 8 in, 1 out]
            n131 = call <vilib>:"CTRE_Phoenix_MotorControl_SelectProfile Slot.vi"("pidLoopIdx"=w229, "slotIdx"=w228, "PhoenixMotorControlDevRef"=w230) -> ()  [unwired: 7 in, 2 out]
            n132 = call <vilib>:"WPI_UtilitiesFRC SendMessageToConsole.vi"("Message"="One Axis Velocity Set\nPress Button 6 to set position") -> ()  [unwired: 14 in, 1 out]
          }
        }
      }
      frame "One_Axis_Velocity_CustomFeedFwd" {
        # "+ 500 RPM"
        n133 = global read "Constants.vi" "Encoder Units\nPer Rotation"() -> (w244:i32)
        n134 = Multiply(x=w234, y=0.25) -> (x*y=w232:dbl)
        n135 = Multiply(x=w235, y=500.0) -> (x*y=w246:dbl)
        n136 = Multiply(x=w246, y=w244) -> (x*y=w243:dbl)
        n137 = Divide(x=w243, y=600.0) -> (x/y=w242:dbl)
        n138 = case shown="\"On\"" w236 {
          tunnel: w240 -> [_ w253]
          tunnel: w239 -> [_ w249]
          tunnel: w242 -> [_ w251]
          tunnel: w232 -> [_ w247]
          frame Default {
          }
          frame "On" {
            w252 = T15 2 items=["PercentOutput"=0, "Position"=1, "Velocity"=2, "Current"=3, "Follower"=5, "MotionProfile"=6, "MotionMagic"=7, "MotionProfileArc"=10, "Disabled"=15] ("Control Mode")
            n139 = call <vilib>:"CTRE_Phoenix_MotorControl_Set.vi"("Demand1"=w247, "DemandType"=T12."DemandType_ArbitraryFeedForward", "Output"=w251, "Control Mode"=w252, "PhoenixMotorControlDevRef"=w253) -> ("PhoenixMotorControlDevRef"=w250:T3)  [unwired: 5 in, 1 out]
            n140 = call <vilib>:"CTRE_Phoenix_MotorControl_Follow.vi"("Master Controller to Follow"=w250, "PhoenixMotorControlDevRef"=w249) -> ()  [unwired: 8 in, 2 out]
          }
        }
        n141 = case shown="True" w237 {
          tunnel: w240 -> [_ w255]
          tunnel: w239 -> [_ w254]
          tunnel: w238 -> [_ _]
          frame False {
          }
          frame True {
            n142 = global read "Constants.vi" "Velocity Slot"() -> (w256:i32)
            n143 = global read "Constants.vi" "PID Primary"() -> (w257:i32)
            n144 = call "Stop Motors.vi"("Talon SRX 2"=w254, "Talon SRX 1"=w255) -> ("Talon SRX 1"=w258:T3)  [unwired: 8 in, 1 out]
            n145 = call <vilib>:"CTRE_Phoenix_MotorControl_SelectProfile Slot.vi"("pidLoopIdx"=w257, "slotIdx"=w256, "PhoenixMotorControlDevRef"=w258) -> ()  [unwired: 7 in, 2 out]
            n146 = call <vilib>:"WPI_UtilitiesFRC SendMessageToConsole.vi"("Message"="One Axis Velocity with Custom Feed Fwd Selected\nPress Button 6 to set position") -> ()  [unwired: 14 in, 1 out]
          }
        }
      }
      frame "Two_Axis_Velocity" {
        # "+ 500 RPM"
        n147 = global read "Constants.vi" "Turn Travel\nUnits Per Rotation"() -> (w262:dbl)
        n148 = global read "Constants.vi" "Encoder Units\nPer Rotation"() -> (w273:i32)
        n149 = Multiply(x=w266, y=w262) -> (x*y=w261:dbl)
        n150 = Multiply(x=w267, y=500.0) -> (x*y=w275:dbl)
        n151 = Multiply(x=w275, y=w273) -> (x*y=w272:dbl)
        n152 = Negate(x=w261) -> (-x=w260:dbl)
        n153 = Divide(x=w272, y=600.0) -> (x/y=w271:dbl)
        n154 = case shown="\"On\"" w268 {
          tunnel: w263 -> [_ w283]
          tunnel: w264 -> [_ w279]
          tunnel: w271 -> [_ w281]
          tunnel: w260 -> [_ w277]
          frame Default {
          }
          frame "On" {
            w282 = T15 2 items=["PercentOutput"=0, "Position"=1, "Velocity"=2, "Current"=3, "Follower"=5, "MotionProfile"=6, "MotionMagic"=7, "MotionProfileArc"=10, "Disabled"=15] ("Control Mode")
            n155 = call <vilib>:"CTRE_Phoenix_MotorControl_Set.vi"("Demand1"=w277, "DemandType"=T12."DemandType_AuxPID", "Output"=w281, "Control Mode"=w282, "PhoenixMotorControlDevRef"=w283) -> ("PhoenixMotorControlDevRef"=w280:T3)  [unwired: 5 in, 1 out]
            n156 = call <vilib>:"CTRE_Phoenix_MotorControl_Follow.vi"("FollowerType"=T13."FollowerType_AuxOutput1", "Master Controller to Follow"=w280, "PhoenixMotorControlDevRef"=w279) -> ()  [unwired: 7 in, 2 out]
          }
        }
        n157 = case shown="True" w269 {
          tunnel: w263 -> [_ w288]
          tunnel: w264 -> [_ w287]
          tunnel: w265 -> [_ _]
          frame False {
          }
          frame True {
            n158 = global read "Constants.vi" "Velocity Slot"() -> (w289:i32)
            n159 = global read "Constants.vi" "PID Primary"() -> (w290:i32)
            n160 = global read "Constants.vi" "Turn Slot"() -> (w286:i32)
            n161 = global read "Constants.vi" "PID Turn"() -> (w284:i32)
            n162 = call "Stop Motors.vi"("Talon SRX 2"=w287, "Talon SRX 1"=w288) -> ("Talon SRX 1"=w291:T3)  [unwired: 8 in, 1 out]
            n163 = call <vilib>:"CTRE_Phoenix_MotorControl_SelectProfile Slot.vi"("pidLoopIdx"=w290, "slotIdx"=w289, "PhoenixMotorControlDevRef"=w291) -> ("PhoenixMotorControlDevRef"=w285:T3)  [unwired: 7 in, 1 out]
            n164 = call <vilib>:"CTRE_Phoenix_MotorControl_SelectProfile Slot.vi"("pidLoopIdx"=w284, "slotIdx"=w286, "PhoenixMotorControlDevRef"=w285) -> ()  [unwired: 7 in, 2 out]
            n165 = call <vilib>:"WPI_UtilitiesFRC SendMessageToConsole.vi"("Message"="Two Axis Velocity\nPress Button 6 to set position") -> ()  [unwired: 14 in, 1 out]
          }
        }
      }
      frame "One_Axis_MotionMagic" {
        n166 = global read "Constants.vi" "Rotations\nTo Travel"() -> (w293:dbl)
        n167 = global read "Constants.vi" "Sensor Units\nPer Rotation"() -> (w301:i32)
        n168 = Multiply(x=w295, y=w293) -> (x*y=w302:dbl)
        n169 = Multiply(x=w302, y=w301) -> (x*y=w294:dbl)
        n170 = case shown="\"On\"" w296 {
          tunnel: w300 -> [_ w307]
          tunnel: w298 -> [_ w303]
          tunnel: w294 -> [_ w305]
          frame Default {
          }
          frame "On" {
            w306 = T15 7 items=["PercentOutput"=0, "Position"=1, "Velocity"=2, "Current"=3, "Follower"=5, "MotionProfile"=6, "MotionMagic"=7, "MotionProfileArc"=10, "Disabled"=15] ("Control Mode")
            n171 = call <vilib>:"CTRE_Phoenix_MotorControl_Set.vi"("Output"=w305, "Control Mode"=w306, "PhoenixMotorControlDevRef"=w307) -> ("PhoenixMotorControlDevRef"=w304:T3)  [unwired: 7 in, 1 out]
            n172 = call <vilib>:"CTRE_Phoenix_MotorControl_Follow.vi"("Master Controller to Follow"=w304, "PhoenixMotorControlDevRef"=w303) -> ()  [unwired: 8 in, 2 out]
          }
        }
        n173 = case shown="True" w297 {
          tunnel: w300 -> [_ w310]
          tunnel: w298 -> [_ w309]
          tunnel: w299 -> [_ w308]
          frame False {
          }
          frame True {
            n174 = call "ZeroSensors.vi"("Pigeon"=w308, "Talon 2"=w309, "Talon 1"=w310) -> ("Talon 2"=w311:T3, "Talon 1"=w312:T3)  [unwired: 6 in, 1 out]
            n175 = global read "Constants.vi" "Motion Profile Slot"() -> (w313:i32)
            n176 = global read "Constants.vi" "PID Primary"() -> (w314:i32)
            n177 = call "Stop Motors.vi"("Talon SRX 2"=w311, "Talon SRX 1"=w312) -> ("Talon SRX 1"=w315:T3)  [unwired: 8 in, 1 out]
            n178 = call <vilib>:"CTRE_Phoenix_MotorControl_SelectProfile Slot.vi"("pidLoopIdx"=w314, "slotIdx"=w313, "PhoenixMotorControlDevRef"=w315) -> ()  [unwired: 7 in, 2 out]
            n179 = call <vilib>:"WPI_UtilitiesFRC SendMessageToConsole.vi"("Message"="One Axis Motion Magic Selected\nPress Button 6 to set position") -> ()  [unwired: 14 in, 1 out]
          }
        }
      }
      frame "One_Axis_MotionMagic_CustomFeedFwd" {
        n180 = global read "Constants.vi" "Rotations\nTo Travel"() -> (w326:dbl)
        n181 = global read "Constants.vi" "Sensor Units\nPer Rotation"() -> (w328:i32)
        n182 = Multiply(x=w319, y=0.25) -> (x*y=w317:dbl)
        n183 = Multiply(x=w325, y=w326) -> (x*y=w329:dbl)
        n184 = Multiply(x=w329, y=w328) -> (x*y=w327:dbl)
        n185 = case shown="\"On\"" w324 {
          tunnel: w320 -> [_ w336]
          tunnel: w321 -> [_ w332]
          tunnel: w327 -> [_ w334]
          tunnel: w317 -> [_ w331]
          frame Default {
          }
          frame "On" {
            w335 = T15 7 items=["PercentOutput"=0, "Position"=1, "Velocity"=2, "Current"=3, "Follower"=5, "MotionProfile"=6, "MotionMagic"=7, "MotionProfileArc"=10, "Disabled"=15] ("Control Mode")
            n186 = call <vilib>:"CTRE_Phoenix_MotorControl_Set.vi"("Demand1"=w331, "DemandType"=T12."DemandType_ArbitraryFeedForward", "Output"=w334, "Control Mode"=w335, "PhoenixMotorControlDevRef"=w336) -> ("PhoenixMotorControlDevRef"=w333:T3)  [unwired: 5 in, 1 out]
            n187 = call <vilib>:"CTRE_Phoenix_MotorControl_Follow.vi"("Master Controller to Follow"=w333, "PhoenixMotorControlDevRef"=w332) -> ()  [unwired: 8 in, 2 out]
          }
        }
        n188 = case shown="True" w323 {
          tunnel: w320 -> [_ w338]
          tunnel: w321 -> [_ w337]
          tunnel: w322 -> [_ _]
          frame False {
          }
          frame True {
            n189 = global read "Constants.vi" "Motion Profile Slot"() -> (w339:i32)
            n190 = global read "Constants.vi" "PID Primary"() -> (w340:i32)
            n191 = call "Stop Motors.vi"("Talon SRX 2"=w337, "Talon SRX 1"=w338) -> ("Talon SRX 1"=w341:T3)  [unwired: 8 in, 1 out]
            n192 = call <vilib>:"CTRE_Phoenix_MotorControl_SelectProfile Slot.vi"("pidLoopIdx"=w340, "slotIdx"=w339, "PhoenixMotorControlDevRef"=w341) -> ()  [unwired: 7 in, 2 out]
            n193 = call <vilib>:"WPI_UtilitiesFRC SendMessageToConsole.vi"("Message"="One Axis Motion Magic with Custom Feed Fwd Selected\nPress Button 6 to set position") -> ()  [unwired: 14 in, 1 out]
          }
        }
      }
      frame "Two_Axis_MotionMagic" {
        n194 = global read "Constants.vi" "Sensor Units\nPer Rotation"() -> (w355:i32)
        n195 = global read "Constants.vi" "Turn Travel\nUnits Per Rotation"() -> (w352:dbl)
        n196 = global read "Constants.vi" "Rotations\nTo Travel"() -> (w354:dbl)
        n197 = Multiply(x=w347, y=w352) -> (x*y=w351:dbl)
        n198 = Multiply(x=w348, y=w355) -> (x*y=w356:dbl)
        n199 = Negate(x=w351) -> (-x=w350:dbl)
        n200 = Multiply(x=w356, y=w354) -> (x*y=w353:dbl)
        n201 = case shown="\"On\"" w349 {
          tunnel: w344 -> [_ w364]
          tunnel: w345 -> [_ w358]
          tunnel: w350 -> [_ w360]
          tunnel: w353 -> [_ w362]
          frame Default {
          }
          frame "On" {
            w363 = T15 7 items=["PercentOutput"=0, "Position"=1, "Velocity"=2, "Current"=3, "Follower"=5, "MotionProfile"=6, "MotionMagic"=7, "MotionProfileArc"=10, "Disabled"=15] ("Control Mode")
            n202 = call <vilib>:"CTRE_Phoenix_MotorControl_Set.vi"("Demand1"=w360, "DemandType"=T12."DemandType_ArbitraryFeedForward", "Output"=w362, "Control Mode"=w363, "PhoenixMotorControlDevRef"=w364) -> ("PhoenixMotorControlDevRef"=w359:T3)  [unwired: 5 in, 1 out]
            n203 = call <vilib>:"CTRE_Phoenix_MotorControl_Follow.vi"("FollowerType"=T13."FollowerType_AuxOutput1", "Master Controller to Follow"=w359, "PhoenixMotorControlDevRef"=w358) -> ()  [unwired: 7 in, 2 out]
          }
        }
        n204 = case shown="True" w343 {
          tunnel: w344 -> [_ w373]
          tunnel: w345 -> [_ w372]
          tunnel: w346 -> [_ w371]
          frame False {
          }
          frame True {
            n205 = global read "Constants.vi" "Motion Profile Slot"() -> (w368:i32)
            n206 = global read "Constants.vi" "PID Primary"() -> (w369:i32)
            n207 = global read "Constants.vi" "Turn Slot"() -> (w367:i32)
            n208 = global read "Constants.vi" "PID Turn"() -> (w366:i32)
            n209 = call "ZeroSensors.vi"("Pigeon"=w371, "Talon 2"=w372, "Talon 1"=w373) -> ("Talon 2"=w374:T3, "Talon 1"=w375:T3)  [unwired: 6 in, 1 out]
            n210 = call "Stop Motors.vi"("Talon SRX 2"=w374, "Talon SRX 1"=w375) -> ("Talon SRX 1"=w370:T3)  [unwired: 8 in, 1 out]
            n211 = call <vilib>:"CTRE_Phoenix_MotorControl_SelectProfile Slot.vi"("pidLoopIdx"=w369, "slotIdx"=w368, "PhoenixMotorControlDevRef"=w370) -> ("PhoenixMotorControlDevRef"=w365:T3)  [unwired: 7 in, 1 out]
            n212 = call <vilib>:"CTRE_Phoenix_MotorControl_SelectProfile Slot.vi"("pidLoopIdx"=w366, "slotIdx"=w367, "PhoenixMotorControlDevRef"=w365) -> ()  [unwired: 7 in, 2 out]
            n213 = call <vilib>:"WPI_UtilitiesFRC SendMessageToConsole.vi"("Message"="Two Axis Motion Magic Selected\nPress Button 6 to set position") -> ()  [unwired: 14 in, 1 out]
          }
        }
      }
      frame "One_Axis_MotionProfile" {
        n214 = Greater Or Equal To 0?(x=w382) -> (x >= 0?=w381:bool)
        n215 = Select(t=i16 1 ("Forward"), s=w381, f=i16 -1) -> (s? t:f=w380:i16)
        n216 = global write "SelectedMotionProfileMode.vi" "Forward"(w380) -> ()
        n217 = global write "SelectedMotionProfileMode.vi" "End Heading"(i16 0 ("End Heading")) -> ()
        n218 = case shown="\"On->Off\"" w383 {
          tunnel: w387 -> [_ w392 w394 w399]
          tunnel: w386 -> [_ w389 _ w398]
          frame Default {
          }
          frame "On" {
            w391 = T15 6 items=["PercentOutput"=0, "Position"=1, "Velocity"=2, "Current"=3, "Follower"=5, "MotionProfile"=6, "MotionMagic"=7, "MotionProfileArc"=10, "Disabled"=15] ("Control Mode")
            n219 = call <vilib>:"CTRE_Phoenix_MotorControl_Set.vi"("Output"=1.0, "Control Mode"=w391, "PhoenixMotorControlDevRef"=w392) -> ("PhoenixMotorControlDevRef"=w390:T3)  [unwired: 7 in, 1 out]
            n220 = call <vilib>:"CTRE_Phoenix_MotorControl_Follow.vi"("Master Controller to Follow"=w390, "PhoenixMotorControlDevRef"=w389) -> ()  [unwired: 8 in, 2 out]
          }
          frame "On->Off" {
            n221 = global write "SelectedMotionProfileMode.vi" "Reset"(TRUE ("Reset")) -> ()
            n222 = call <vilib>:"CTRE_Phoenix_MotorControl_ClearMotionProfileHasUnderrun.vi"("PhoenixMotorControlDevRef"=w394) -> ("error out"=w395:errorcluster, "PhoenixMotorControlDevRef"=w396:T3)  [unwired: 9 in]
            n223 = call <vilib>:"CTRE_Phoenix_MotorControl_ClearMotionProfileTrajectories.vi"("PhoenixMotorControlDevRef"=w396, "error in"=w395) -> ()  [unwired: 12 in, 2 out]
          }
          frame "Off" {
            w397 = T15 6 items=["PercentOutput"=0, "Position"=1, "Velocity"=2, "Current"=3, "Follower"=5, "MotionProfile"=6, "MotionMagic"=7, "MotionProfileArc"=10, "Disabled"=15] ("Control Mode")
            n224 = call <vilib>:"CTRE_Phoenix_MotorControl_Set.vi"("Output"=0.0, "Control Mode"=w397, "PhoenixMotorControlDevRef"=w399) -> ("PhoenixMotorControlDevRef"=w401:T3)  [unwired: 7 in, 1 out]
            n225 = call <vilib>:"CTRE_Phoenix_MotorControl_Follow.vi"("Master Controller to Follow"=w401, "PhoenixMotorControlDevRef"=w398) -> ()  [unwired: 8 in, 2 out]
          }
        }
        n226 = case shown="True" w384 {
          tunnel: w387 -> [_ w404]
          tunnel: w386 -> [_ w403]
          tunnel: w385 -> [_ w402]
          frame False {
          }
          frame True {
            n227 = call "ZeroSensors.vi"("Pigeon"=w402, "Talon 2"=w403, "Talon 1"=w404) -> ("Talon 2"=w405:T3, "Talon 1"=w406:T3)  [unwired: 6 in, 1 out]
            n228 = global read "Constants.vi" "Motion Profile Slot"() -> (w407:i32)
            n229 = global read "Constants.vi" "PID Primary"() -> (w408:i32)
            n230 = call "Stop Motors.vi"("Talon SRX 2"=w405, "Talon SRX 1"=w406) -> ("Talon SRX 1"=w409:T3)  [unwired: 8 in, 1 out]
            n231 = call <vilib>:"CTRE_Phoenix_MotorControl_SelectProfile Slot.vi"("pidLoopIdx"=w408, "slotIdx"=w407, "PhoenixMotorControlDevRef"=w409) -> ()  [unwired: 7 in, 2 out]
            n232 = call <vilib>:"WPI_UtilitiesFRC SendMessageToConsole.vi"("Message"="One Axis Motion Profile Selected\nPress Button 6 to fire the profile") -> ()  [unwired: 14 in, 1 out]
          }
        }
      }
      frame "One_Axis_MotionProfile_CustomFeedFwd" {
        n233 = Greater Or Equal To 0?(x=w414) -> (x >= 0?=w424:bool)
        n234 = Select(t=i16 1 ("Forward"), s=w424, f=i16 -1) -> (s? t:f=w423:i16)
        n235 = global write "SelectedMotionProfileMode.vi" "Forward"(w423) -> ()
        n236 = Multiply(x=w411, y=0.25) -> (x*y=w413:dbl)
        n237 = global write "SelectedMotionProfileMode.vi" "End Heading"(i16 0 ("End Heading")) -> ()
        n238 = case shown="\"On->Off\"" w415 {
          tunnel: w419 -> [_ w431 w434 w440]
          tunnel: w418 -> [_ w428 _ w439]
          tunnel: w413 -> [_ w425 _ _]
          frame Default {
          }
          frame "On" {
            w430 = T15 6 items=["PercentOutput"=0, "Position"=1, "Velocity"=2, "Current"=3, "Follower"=5, "MotionProfile"=6, "MotionMagic"=7, "MotionProfileArc"=10, "Disabled"=15] ("Control Mode")
            n239 = call <vilib>:"CTRE_Phoenix_MotorControl_Set.vi"("Demand1"=w425, "DemandType"=T12."DemandType_ArbitraryFeedForward", "Output"=1.0, "Control Mode"=w430, "PhoenixMotorControlDevRef"=w431) -> ("PhoenixMotorControlDevRef"=w429:T3)  [unwired: 5 in, 1 out]
            n240 = call <vilib>:"CTRE_Phoenix_MotorControl_Follow.vi"("Master Controller to Follow"=w429, "PhoenixMotorControlDevRef"=w428) -> ()  [unwired: 8 in, 2 out]
          }
          frame "On->Off" {
            n241 = global write "SelectedMotionProfileMode.vi" "Reset"(TRUE ("Reset")) -> ()
            n242 = call <vilib>:"CTRE_Phoenix_MotorControl_ClearMotionProfileHasUnderrun.vi"("PhoenixMotorControlDevRef"=w434) -> ("error out"=w435:errorcluster, "PhoenixMotorControlDevRef"=w433:T3)  [unwired: 9 in]
            n243 = call <vilib>:"CTRE_Phoenix_MotorControl_ClearMotionProfileTrajectories.vi"("PhoenixMotorControlDevRef"=w433, "error in"=w435) -> ()  [unwired: 12 in, 2 out]
          }
          frame "Off" {
            w436 = 0.0 ("Output")
            w438 = T15 6 items=["PercentOutput"=0, "Position"=1, "Velocity"=2, "Current"=3, "Follower"=5, "MotionProfile"=6, "MotionMagic"=7, "MotionProfileArc"=10, "Disabled"=15] ("Control Mode")
            n244 = call <vilib>:"CTRE_Phoenix_MotorControl_Set.vi"("Demand1"=w436, "DemandType"=T12."DemandType_ArbitraryFeedForward", "Output"=w436, "Control Mode"=w438, "PhoenixMotorControlDevRef"=w440) -> ("PhoenixMotorControlDevRef"=w441:T3)  [unwired: 5 in, 1 out]
            n245 = call <vilib>:"CTRE_Phoenix_MotorControl_Follow.vi"("Master Controller to Follow"=w441, "PhoenixMotorControlDevRef"=w439) -> ()  [unwired: 8 in, 2 out]
          }
        }
        n246 = case shown="True" w416 {
          tunnel: w419 -> [_ w444]
          tunnel: w418 -> [_ w443]
          tunnel: w417 -> [_ w442]
          frame False {
          }
          frame True {
            n247 = call "ZeroSensors.vi"("Pigeon"=w442, "Talon 2"=w443, "Talon 1"=w444) -> ("Talon 2"=w445:T3, "Talon 1"=w446:T3)  [unwired: 6 in, 1 out]
            n248 = global read "Constants.vi" "Motion Profile Slot"() -> (w447:i32)
            n249 = global read "Constants.vi" "PID Primary"() -> (w448:i32)
            n250 = call "Stop Motors.vi"("Talon SRX 2"=w445, "Talon SRX 1"=w446) -> ("Talon SRX 1"=w449:T3)  [unwired: 8 in, 1 out]
            n251 = call <vilib>:"CTRE_Phoenix_MotorControl_SelectProfile Slot.vi"("pidLoopIdx"=w448, "slotIdx"=w447, "PhoenixMotorControlDevRef"=w449) -> ()  [unwired: 7 in, 2 out]
            n252 = call <vilib>:"WPI_UtilitiesFRC SendMessageToConsole.vi"("Message"="One Axis Motion Profile with Custom Feed Fwd Selected\nPress Button 6 to fire the profile") -> ()  [unwired: 14 in, 1 out]
          }
        }
      }
      frame "Two_Axis_MotionProfile" {
        n253 = global read "Constants.vi" "Turn Travel\nUnits Per Rotation"() -> (w453:dbl)
        n254 = Greater Or Equal To 0?(x=w455) -> (x >= 0?=w464:bool)
        n255 = Select(t=i16 1 ("Forward"), s=w464, f=i16 -1) -> (s? t:f=w463:i16)
        n256 = global write "SelectedMotionProfileMode.vi" "Forward"(w463) -> ()
        n257 = Multiply(x=w454, y=w453) -> (x*y=w452:dbl)
        n258 = Negate(x=w452) -> (-x=w451:dbl)
        n259 = case shown="\"On\"" w456 {
          tunnel: w457 -> [_ w471 w473 w480]
          tunnel: w458 -> [_ w468 _ w479]
          frame Default {
          }
          frame "On" {
            w470 = T15 10 items=["PercentOutput"=0, "Position"=1, "Velocity"=2, "Current"=3, "Follower"=5, "MotionProfile"=6, "MotionMagic"=7, "MotionProfileArc"=10, "Disabled"=15] ("Control Mode")
            n260 = call <vilib>:"CTRE_Phoenix_MotorControl_Set.vi"("Demand1"=0.0, "DemandType"=T12."DemandType_ArbitraryFeedForward", "Output"=1.0, "Control Mode"=w470, "PhoenixMotorControlDevRef"=w471) -> ("PhoenixMotorControlDevRef"=w469:T3)  [unwired: 5 in, 1 out]
            n261 = call <vilib>:"CTRE_Phoenix_MotorControl_Follow.vi"("Master Controller to Follow"=w469, "PhoenixMotorControlDevRef"=w468) -> ()  [unwired: 8 in, 2 out]
          }
          frame "On->Off" {
            n262 = global write "SelectedMotionProfileMode.vi" "Reset"(TRUE ("Reset")) -> ()
            n263 = call <vilib>:"CTRE_Phoenix_MotorControl_ClearMotionProfileHasUnderrun.vi"("PhoenixMotorControlDevRef"=w473) -> ("error out"=w475:errorcluster, "PhoenixMotorControlDevRef"=w474:T3)  [unwired: 9 in]
            n264 = call <vilib>:"CTRE_Phoenix_MotorControl_ClearMotionProfileTrajectories.vi"("PhoenixMotorControlDevRef"=w474, "error in"=w475) -> ()  [unwired: 12 in, 2 out]
          }
          frame "Off" {
            w476 = 0.0 ("Output")
            w478 = T15 6 items=["PercentOutput"=0, "Position"=1, "Velocity"=2, "Current"=3, "Follower"=5, "MotionProfile"=6, "MotionMagic"=7, "MotionProfileArc"=10, "Disabled"=15] ("Control Mode")
            n265 = call <vilib>:"CTRE_Phoenix_MotorControl_Set.vi"("Demand1"=w476, "DemandType"=T12."DemandType_ArbitraryFeedForward", "Output"=w476, "Control Mode"=w478, "PhoenixMotorControlDevRef"=w480) -> ("PhoenixMotorControlDevRef"=w481:T3)  [unwired: 5 in, 1 out]
            n266 = call <vilib>:"CTRE_Phoenix_MotorControl_Follow.vi"("Master Controller to Follow"=w481, "PhoenixMotorControlDevRef"=w479) -> ()  [unwired: 8 in, 2 out]
          }
        }
        n267 = global write "SelectedMotionProfileMode.vi" "End Heading"(w451) -> ()
        n268 = case shown="True" w460 {
          tunnel: w457 -> [_ w484]
          tunnel: w458 -> [_ w483]
          tunnel: w459 -> [_ w482]
          frame False {
          }
          frame True {
            n269 = call "ZeroSensors.vi"("Pigeon"=w482, "Talon 2"=w483, "Talon 1"=w484) -> ("Talon 2"=w485:T3, "Talon 1"=w486:T3)  [unwired: 6 in, 1 out]
            n270 = global read "Constants.vi" "Motion Profile Slot"() -> (w487:i32)
            n271 = global read "Constants.vi" "PID Primary"() -> (w488:i32)
            n272 = call "Stop Motors.vi"("Talon SRX 2"=w485, "Talon SRX 1"=w486) -> ("Talon SRX 1"=w489:T3)  [unwired: 8 in, 1 out]
            n273 = call <vilib>:"CTRE_Phoenix_MotorControl_SelectProfile Slot.vi"("pidLoopIdx"=w488, "slotIdx"=w487, "PhoenixMotorControlDevRef"=w489) -> ()  [unwired: 7 in, 2 out]
            n274 = call <vilib>:"WPI_UtilitiesFRC SendMessageToConsole.vi"("Message"="Two Axis Motion Profile Selected\nPress Button 6 to fire the profile") -> ()  [unwired: 14 in, 1 out]
          }
        }
      }
      frame "Two_Axis_MotionProfile_CustomFeedFwd" {
        n275 = global read "Constants.vi" "Turn Travel\nUnits Per Rotation"() -> (w503:dbl)
        n276 = Greater Or Equal To 0?(x=w495) -> (x >= 0?=w507:bool)
        n277 = Select(t=i16 1 ("Forward"), s=w507, f=i16 -1) -> (s? t:f=w506:i16)
        n278 = Multiply(x=w493, y=0.25) -> (x*y=w491:dbl)
        n279 = global write "SelectedMotionProfileMode.vi" "Forward"(w506) -> ()
        n280 = Multiply(x=w494, y=w503) -> (x*y=w502:dbl)
        n281 = Negate(x=w502) -> (-x=w501:dbl)
        n282 = case shown="\"On\"" w496 {
          tunnel: w500 -> [_ w515 w517 w524]
          tunnel: w499 -> [_ w512 _ w523]
          tunnel: w491 -> [_ w509 _ _]
          frame Default {
          }
          frame "On" {
            w514 = T15 10 items=["PercentOutput"=0, "Position"=1, "Velocity"=2, "Current"=3, "Follower"=5, "MotionProfile"=6, "MotionMagic"=7, "MotionProfileArc"=10, "Disabled"=15] ("Control Mode")
            n283 = call <vilib>:"CTRE_Phoenix_MotorControl_Set.vi"("Demand1"=w509, "DemandType"=T12."DemandType_ArbitraryFeedForward", "Output"=1.0, "Control Mode"=w514, "PhoenixMotorControlDevRef"=w515) -> ("PhoenixMotorControlDevRef"=w513:T3)  [unwired: 5 in, 1 out]
            n284 = call <vilib>:"CTRE_Phoenix_MotorControl_Follow.vi"("FollowerType"=T13."FollowerType_AuxOutput1", "Master Controller to Follow"=w513, "PhoenixMotorControlDevRef"=w512) -> ()  [unwired: 7 in, 2 out]
          }
          frame "On->Off" {
            n285 = global write "SelectedMotionProfileMode.vi" "Reset"(TRUE ("Reset")) -> ()
            n286 = call <vilib>:"CTRE_Phoenix_MotorControl_ClearMotionProfileHasUnderrun.vi"("PhoenixMotorControlDevRef"=w517) -> ("error out"=w519:errorcluster, "PhoenixMotorControlDevRef"=w518:T3)  [unwired: 9 in]
            n287 = call <vilib>:"CTRE_Phoenix_MotorControl_ClearMotionProfileTrajectories.vi"("PhoenixMotorControlDevRef"=w518, "error in"=w519) -> ()  [unwired: 12 in, 2 out]
          }
          frame "Off" {
            w520 = 0.0 ("Output")
            w522 = T15 6 items=["PercentOutput"=0, "Position"=1, "Velocity"=2, "Current"=3, "Follower"=5, "MotionProfile"=6, "MotionMagic"=7, "MotionProfileArc"=10, "Disabled"=15] ("Control Mode")
            n288 = call <vilib>:"CTRE_Phoenix_MotorControl_Set.vi"("Demand1"=w520, "DemandType"=T12."DemandType_ArbitraryFeedForward", "Output"=w520, "Control Mode"=w522, "PhoenixMotorControlDevRef"=w524) -> ("PhoenixMotorControlDevRef"=w525:T3)  [unwired: 5 in, 1 out]
            n289 = call <vilib>:"CTRE_Phoenix_MotorControl_Follow.vi"("Master Controller to Follow"=w525, "PhoenixMotorControlDevRef"=w523) -> ()  [unwired: 8 in, 2 out]
          }
        }
        n290 = global write "SelectedMotionProfileMode.vi" "End Heading"(w501) -> ()
        n291 = case shown="True" w497 {
          tunnel: w500 -> [_ w528]
          tunnel: w499 -> [_ w527]
          tunnel: w498 -> [_ w526]
          frame False {
          }
          frame True {
            n292 = call "ZeroSensors.vi"("Pigeon"=w526, "Talon 2"=w527, "Talon 1"=w528) -> ("Talon 2"=w529:T3, "Talon 1"=w530:T3)  [unwired: 6 in, 1 out]
            n293 = global read "Constants.vi" "Motion Profile Slot"() -> (w531:i32)
            n294 = global read "Constants.vi" "PID Primary"() -> (w532:i32)
            n295 = call "Stop Motors.vi"("Talon SRX 2"=w529, "Talon SRX 1"=w530) -> ("Talon SRX 1"=w533:T3)  [unwired: 8 in, 1 out]
            n296 = call <vilib>:"CTRE_Phoenix_MotorControl_SelectProfile Slot.vi"("pidLoopIdx"=w532, "slotIdx"=w531, "PhoenixMotorControlDevRef"=w533) -> ()  [unwired: 7 in, 2 out]
            n297 = call <vilib>:"WPI_UtilitiesFRC SendMessageToConsole.vi"("Message"="Two Axis Motion Profile With Custom Feed ForwardSelected\nPress Button 6 to fire the profile") -> ()  [unwired: 14 in, 1 out]
          }
        }
      }
    }
  }
  n298 = while {
    tunnel: w13 -> [w589]
    shift-right: [w565] -> _
    shift-left: _ -> [w588]
    tunnel: w12 -> [w569]
    tunnel: w5 -> [w568]
    shift-right: [w573] -> _
    shift-left: _ -> [w572]
    stop <- FALSE stop-if-true
    # "Track loop time"
    # "When in PercentOutput, report fault"
    # "Check if sensor is out of phase, this is not necessary and can be removed"
    # "Call Motion Prof once per loop to ensure it can keep pace with motion profile executer in Talon SRX.  Also lets poll if we can insert the next point.  Also compare cursor with total count to see if we still need to send another point."
    # "Instrument our signals  to front panel"
    # "Point cursor"
    # "Total Count"
    # "If our cursor is less than total and Talon can fit next point, send it."
    # "If we have more points to insert, and Talon can fit one more, insert that point"
    # "5 ms tasks go here, don't count loops, and don't ever stop."
    n299 = Wait (ms)(milliseconds to wait=u32 5) -> ()  [unwired: 1 out]
    n300 = call <vilib>:"CTRE_Phoenix_MotorControl_GetActiveTrajectory.vi"("PhoenixMotorControlDevRef"=w568) -> ("Position (Sensor Units)"=→"Mot Prof Active Position":i32, "Velocity (Sensor Units per 100 ms)"=→"Mot Prof Active Velocity":i32)  [unwired: 10 in, 3 out]
    n301 = call <vilib>:"CTRE_Phoenix_MotorControl_ProcessMotionProfileBuffer.vi"("PhoenixMotorControlDevRef"=w568) -> ("PhoenixMotorControlDevRef"=w581:T3)  [unwired: 13 in, 1 out]
    n302 = call <vilib>:"CTRE_Phoenix_MotorControl_GetMotionProfileStatus.vi"("PhoenixMotorControlDevRef"=w581) -> ("Motion Profile Status"=w583:T16, "PhoenixMotorControlDevRef"=w585:T3)  [unwired: 8 in, 1 out]
    n303 = Unbundle By Name(w583) -> ("Bottom Buffer Count"=→"Btm Mot Prof Count":i32, "Top Buffer Count"=→"Top Mot Prof Count":i32, "Top Buffer Remaining"=w582:i32, "Has Underrun?"=→"Mot Prof  Has Under Run":bool, "Is Underrun?"=→"Mot Prof  Is Under Run":bool, "Active Point Valid?"=→"Mot Prof Active Is Valid":bool, "Is Last?"=→"Mot Prof Active Is Last":bool)
    n304 = Greater Than 0?(x=w582) -> (x > 0?=w584:bool)
    n305 = Tick Count (ms)() -> (millisecond timer value=w573:u32)
    n306 = Subtract(x=w573, y=w572) -> (x-y=→"Loop Time":u32)
    n307 = Greater Or Equal?(x=w569, y=w588) -> (x >= y?=w586:bool)
    n308 = And(x=w584, y=w586) -> (x .and. y?=w587:bool)
    n309 = case shown="True" w587 {
      tunnel: w589 -> [_ w603]
      tunnel: [w595 w617] -> w567
      tunnel: w588 -> [w595 w618]
      tunnel: w569 -> [_ w602]
      tunnel: w585 -> [_ w616]
      frame False {
      }
      frame True {
        w605 = T17 0 items=["TrajectoryDuration_0ms"=0, "TrajectoryDuration_5ms"=5, "TrajectoryDuration_10ms"=10, "TrajectoryDuration_20ms"=20, "TrajectoryDuration_30ms"=30, "TrajectoryDuration_40ms"=40, "TrajectoryDuration_50ms"=50, "TrajectoryDuration_100ms"=100] ("durationMs")
        # "Create a Trajector Point and fill it in.\nDuration, Vel, and Pos are copied from the csv row.  Slot is hardcoded to match the roboRIO web-based config.  IsLast is true for the last point.  ZeroPosition is true for the first point to auto clear the sensor position."
        n310 = Equal To 0?(x=w618) -> (x = 0?=w614:bool)
        n311 = Index Array(array=w603, index (row)=w618) -> (element=w619:dbl[])  [unwired: 1 in]
        n312 = Add(x=u32 1, y=w618) -> (x+y=w617:u32)
        n313 = Index Array(array=w619) -> (element #1=w611:dbl, element #2=w609:dbl)  [unwired: 3 in, 1 out]
        n314 = Greater Or Equal?(x=w617, y=w602) -> (x >= y?=w613:bool)
        n315 = Multiply(x=-4096.0, y=w611) -> (x*y=w599:dbl)
        n316 = Multiply(x=-4096.0, y=w609) -> (x*y=w607:dbl)
        n317 = Divide(x=w607, y=10.0) -> (x/y=w606:dbl)
        n318 = Index Array(array=w603, index (row)=w602, index (col)=0 ("disabled index (col)")) -> (element=w600:dbl)
        n319 = global read "SelectedMotionProfileMode.vi" "End Heading"() -> (w597:dbl)
        n320 = Divide(x=w599, y=w600) -> (x/y=w598:dbl)
        n321 = Multiply(x=w597, y=w598) -> (x*y=w596:dbl)
        n322 = call <vilib>:"CTRE_Phoenix_MotorControl_PushMotionProfileTrajectory.vi"("PhoenixMotorControlDevRef"=w616, "profileSlotSelect1"=0, "durationMs"=w605, "position"=w599, "velocity"=w606, "auxiliaryPos"=w596, "profileSlotSelect0"=0, "isLastPoint?"=w613, "Zero Position?"=w614) -> ()  [unwired: 5 in, 2 out]
      }
    }
    n323 = global read "SelectedMotionProfileMode.vi" "Reset"() -> (w566:bool)
    n324 = case shown="True" w566 {
      tunnel: w567 -> [w592 _]
      tunnel: [w592 u32 0] -> w565
      frame False {
      }
      frame True {
        n325 = global write "SelectedMotionProfileMode.vi" "Reset"(FALSE ("Reset")) -> ()
      }
    }
  }
  n326 = call-poly <vilib>:"Read Delimited Spreadsheet.vi"() -> ()  [unwired: 10 in, 6 out]
